vi "Lab Panel V5.23.vi"() -> ()   [LabVIEW 2013] (continued)
                          tunnel: w5914 -> [w5942 w5945]
                          tunnel: [w5942 w5944] -> w5912
                          frame False {
                          }
                          frame True {
                            n3204 = Multiply(x=w5946, y=w5945) -> (x*y=w5944:dbl)
                            n3205 = Multiply(x=w5946, y=w5948) -> (x*y=w5947:dbl)
                          }
                        }
                        n3206 = local read "SIG LAB04-2"() -> (w5931:T2)
                        n3207 = local read "SIG LAB04-1"() -> (w5933:T2)
                        n3208 = Bundle By Name(cluster=w5933, "Tmp Live"=w5913, "Tmp Neut"=w5912) -> (w5932:T2)
                        n3209 = Bundle By Name(cluster=w5931, "Tmp Live"=w5909, "Tmp Neut"=w5908) -> (w5930:T2)
                        n3210 = local write "SIG LAB04-1"(w5932) -> ()
                        n3211 = local write "SIG LAB04-2"(w5930) -> ()
                      }
                      frame 5.. {
                        n3212 = case shown="False" w5963 {
                          tunnel: [w5994 w5995] -> w5979
                          tunnel: w5962 -> [_ w5995]
                          frame False {
                            n3213 = local read "CAL LAB05"() -> (w5994:T14)
                          }
                          frame True {
                          }
                        }
                        n3214 = local read "LAB05 TEMP"() -> (w5969:T12)
                        n3215 = local read "TEMP LA05"() -> (w5970:T9)
                        n3216 = call "sub vi - temperature delay v3.vi"("2-run"=w5951, "1-run"=w5952, "temp values IN"=w5970, "temp signals"=w5969) -> ("T2-N"=w5965:dbl, "T2-L"=w5966:dbl, "T1-N"=w5967:dbl, "T1-L"=w5968:dbl, "temp values OUT"=w5964:T44)  [unwired: 3 in]
                        n3217 = local write "TEMP LA05"(w5964) -> ()
                        n3218 = Unbundle By Name(w5979) -> ("1 (TL) cal"=w5971:dbl, "1 (TN) cal"=w5974:dbl, "2 (TL) cal"=w5973:dbl, "2 (TN) cal"=w5972:dbl)  [unwired: 6 out]
                        n3219 = Multiply(x=w5968, y=w5971) -> (x*y=w5960:dbl)
                        n3220 = Multiply(x=w5967, y=w5974) -> (x*y=w5959:dbl)
                        n3221 = Multiply(x=w5966, y=w5973) -> (x*y=w5956:dbl)
                        n3222 = Multiply(x=w5965, y=w5972) -> (x*y=w5955:dbl)
                        n3223 = case shown="True" w5951 {
                          tunnel: w5956 -> [w5981 w5986]
                          tunnel: w5961 -> [_ w5984]
                          tunnel: [w5981 w5985] -> w5954
                          tunnel: w5955 -> [w5980 w5983]
                          tunnel: [w5980 w5982] -> w5953
                          frame False {
                          }
                          frame True {
                            n3224 = Multiply(x=w5984, y=w5983) -> (x*y=w5982:dbl)
                            n3225 = Multiply(x=w5984, y=w5986) -> (x*y=w5985:dbl)
                          }
                        }
                        n3226 = case shown="True" w5952 {
                          tunnel: w5960 -> [w5988 w5993]
                          tunnel: w5961 -> [_ w5991]
                          tunnel: [w5988 w5992] -> w5958
                          tunnel: w5959 -> [w5987 w5990]
                          tunnel: [w5987 w5989] -> w5957
                          frame False {
                          }
                          frame True {
                            n3227 = Multiply(x=w5991, y=w5990) -> (x*y=w5989:dbl)
                            n3228 = Multiply(x=w5991, y=w5993) -> (x*y=w5992:dbl)
                          }
                        }
                        n3229 = local read "SIG LAB05-1"() -> (w5978:T2)
                        n3230 = Bundle By Name(cluster=w5978, "Tmp Live"=w5958, "Tmp Neut"=w5957) -> (w5977:T2)
                        n3231 = local read "SIG LAB05-2"() -> (w5976:T2)
                        n3232 = Bundle By Name(cluster=w5976, "Tmp Live"=w5954, "Tmp Neut"=w5953) -> (w5975:T2)
                        n3233 = local write "SIG LAB05-1"(w5977) -> ()
                        n3234 = local write "SIG LAB05-2"(w5975) -> ()
                      }
                    }
                  }
                }
              }
            }
          }
          frame #20 {
            # "write data to display panel"
            n3235 = global write "Global display 1.vi" "TEST 5-2"(w6030) -> ()
            n3236 = global write "Global display 1.vi" "TEST 4-2"(w6032) -> ()
            n3237 = global write "Global display 1.vi" "TEST 1-2"(w6038) -> ()
            n3238 = global write "Global display 1.vi" "TEST 3-1"(w6035) -> ()
            n3239 = global write "Global display 1.vi" "TEST 5-1"(w6031) -> ()
            n3240 = global write "Global display 1.vi" "TEST 1-1"(w6039) -> ()
            n3241 = global write "Global display 1.vi" "TEST 3-2"(w6034) -> ()
            n3242 = global write "Global display 1.vi" "TEST 4-1"(w6033) -> ()
            n3243 = global write "Global display 1.vi" "TEST 2-2"(w6036) -> ()
            n3244 = global write "Global display 1.vi" "TEST 2-1"(w6037) -> ()
            n3245 = global read "Global display 3.vi" "log 1-1"() -> (→"LOG LAB01-1":string)
            n3246 = global read "Global display 3.vi" "log 3-1"() -> (→"LOG LAB03-1":string)
            n3247 = global read "Global display 3.vi" "log 1-2"() -> (→"LOG LAB01-2":string)
            n3248 = property on="Tab Control 2" class="TabCtl (strict)"() -> ("Pages"=w6029:refnum<vi>[])  [unwired: 2 in, 2 out]
            n3249 = global read "Global display 3.vi" "log 2-1"() -> (→"LOG LAB02-1":string)
            n3250 = global read "Global display 3.vi" "log 2-2"() -> (→"LOG LAB02-2":string)
            n3251 = global read "Global display 3.vi" "log 4-2"() -> (→"LOG LAB04-2":string)
            n3252 = global read "Global display 3.vi" "log 5-2"() -> (→"LOG LAB05-2":string)
            n3253 = global read "Global display 3.vi" "log 5-1"() -> (→"LOG LAB05-1":string)
            n3254 = global read "Global display 3.vi" "log 4-1"() -> (→"LOG LAB04-1":string)
            n3255 = global read "Global display 3.vi" "log 3-2"() -> (→"LOG LAB03-2":string)
            n3256 = Index Array(array=w6029, index=8) -> (element=w6027:refnum<vi>)
            n3257 = property class="Page"(reference=w6027) -> ("PageVis"=w6026:bool)  [unwired: 1 in, 2 out]
            n3258 = global write "Global display 3.vi" "admin"(w6026) -> ()
            n3259 = local read "O/I  LAB05-2"() -> (w6080:bool)
            n3260 = local read "O/I  LAB05-1"() -> (w6081:bool)
            n3261 = local read "O/I  LAB03-2"() -> (w6084:bool)
            n3262 = local read "O/I  LAB04-2"() -> (w6082:bool)
            n3263 = local read "O/I  LAB04-1"() -> (w6083:bool)
            n3264 = local read "O/I  LAB03-1"() -> (w6085:bool)
            n3265 = local read "O/I  LAB01-2"() -> (w6088:bool)
            n3266 = local read "O/I  LAB01-1"() -> (w6089:bool)
            n3267 = local read "O/I  LAB02-1"() -> (w6087:bool)
            n3268 = local read "O/I  LAB02-2"() -> (w6086:bool)
            n3269 = global write "Global display 1.vi" "5-2 O/F"(w6080) -> ()
            n3270 = global write "Global display 1.vi" "5-1 O/F"(w6081) -> ()
            n3271 = global write "Global display 1.vi" "4-1 O/F"(w6083) -> ()
            n3272 = global write "Global display 1.vi" "4-2 O/F"(w6082) -> ()
            n3273 = global write "Global display 1.vi" "3-2 O/F"(w6084) -> ()
            n3274 = global write "Global display 1.vi" "3-1 O/F"(w6085) -> ()
            n3275 = global write "Global display 1.vi" "2-2 O/F"(w6086) -> ()
            n3276 = global write "Global display 1.vi" "2-1 O/F"(w6087) -> ()
            n3277 = global write "Global display 1.vi" "1-2 O/F"(w6088) -> ()
            n3278 = global write "Global display 1.vi" "1-1 O/F"(w6089) -> ()
            n3279 = local read "TEMP START LAB02-2"() -> (w6012:cluster{"TL":dbl, "TN":dbl})
            n3280 = local read "run lab05-2"() -> (w6070:bool)
            n3281 = local read "TEMP START LAB01-2"() -> (w6014:cluster{"TL":dbl, "TN":dbl})
            n3282 = local read "TEMP START LAB02-1"() -> (w6013:cluster{"TL":dbl, "TN":dbl})
            n3283 = local read "TEMP START LAB04-1"() -> (w6009:cluster{"TL":dbl, "TN":dbl})
            n3284 = local read "TEMP START LAB04-2"() -> (w6008:cluster{"TL":dbl, "TN":dbl})
            n3285 = local read "run lab04-1"() -> (w6073:bool)
            n3286 = local read "run lab04-2"() -> (w6072:bool)
            n3287 = local read "run lab05-1"() -> (w6071:bool)
            n3288 = local read "TEMP START LAB01-1"() -> (w6015:cluster{"TL":dbl, "TN":dbl})
            n3289 = local read "TEMP START LAB05-2"() -> (w6006:cluster{"TL":dbl, "TN":dbl})
            n3290 = local read "TEMP START LAB05-1"() -> (w6007:cluster{"TL":dbl, "TN":dbl})
            n3291 = local read "run lab03-2"() -> (w6074:bool)
            n3292 = local read "TEMP START LAB03-2"() -> (w6010:cluster{"TL":dbl, "TN":dbl})
            n3293 = local read "TEMP START LAB03-1"() -> (w6011:cluster{"TL":dbl, "TN":dbl})
            n3294 = local read "run lab02-1"() -> (w6077:bool)
            n3295 = local read "run lab03-1"() -> (w6075:bool)
            n3296 = local read "run lab01-2"() -> (w6078:bool)
            n3297 = local read "run lab02-2"() -> (w6076:bool)
            n3298 = local read "run lab01-1"() -> (w6079:bool)
            n3299 = global write "Global display 1.vi" "5-2 R/S"(w6070) -> ()
            n3300 = global write "Global display 1.vi" "5-1 R/S"(w6071) -> ()
            n3301 = global write "Global display 1.vi" "4-2 R/S"(w6072) -> ()
            n3302 = global write "Global display 1.vi" "4-1 R/S"(w6073) -> ()
            n3303 = global write "Global display 1.vi" "3-2 R/S"(w6074) -> ()
            n3304 = global write "Global display 1.vi" "1-2 R/S"(w6078) -> ()
            n3305 = global write "Global display 1.vi" "2-1 R/S"(w6077) -> ()
            n3306 = global write "Global display 1.vi" "3-1 R/S"(w6075) -> ()
            n3307 = global write "Global display 1.vi" "2-2 R/S"(w6076) -> ()
            n3308 = global write "Global display 1.vi" "1-1 R/S"(w6079) -> ()
            n3309 = global write "Global display 3.vi" "TEMP ST 05-2"(w6006) -> ()
            n3310 = global write "Global display 3.vi" "TEMP ST 05-1"(w6007) -> ()
            n3311 = global write "Global display 3.vi" "TEMP ST 03-2"(w6010) -> ()
            n3312 = global write "Global display 3.vi" "TEMP ST 04-2"(w6008) -> ()
            n3313 = global write "Global display 3.vi" "TEMP ST 01-1"(w6015) -> ()
            n3314 = global write "Global display 3.vi" "TEMP ST 01-2"(w6014) -> ()
            n3315 = global write "Global display 3.vi" "TEMP ST 04-1"(w6009) -> ()
            n3316 = global write "Global display 3.vi" "TEMP ST 02-1"(w6013) -> ()
            n3317 = global write "Global display 3.vi" "TEMP ST 02-2"(w6012) -> ()
            n3318 = global write "Global display 3.vi" "TEMP ST 03-1"(w6011) -> ()
            n3319 = local read "DISP LAB04-2"() -> (w6062:T4)
            n3320 = local read "DISP LAB05-1"() -> (w6061:T4)
            n3321 = local read "DISP LAB04-1"() -> (w6063:T4)
            n3322 = local read "DISP LAB05-2"() -> (w6060:T4)
            n3323 = local read "DISP LAB03-1"() -> (w6065:T4)
            n3324 = local read "DISP LAB03-2"() -> (w6064:T4)
            n3325 = local read "DISP LAB01-2"() -> (w6068:T4)
            n3326 = local read "DISP LAB02-1"() -> (w6067:T4)
            n3327 = local read "DISP LAB02-2"() -> (w6066:T4)
            n3328 = local read "DISP LAB01-1"() -> (w6069:T4)
            n3329 = local read "TEMP RISE LAB05-1"() -> (w5997:cluster{"TL":dbl, "TN":dbl})
            n3330 = local read "TEMP RISE LAB05-2"() -> (w5996:cluster{"TL":dbl, "TN":dbl})
            n3331 = local read "TEMP RISE LAB04-2"() -> (w5998:cluster{"TL":dbl, "TN":dbl})
            n3332 = local read "TEMP RISE LAB04-1"() -> (w5999:cluster{"TL":dbl, "TN":dbl})
            n3333 = local read "TEMP RISE LAB03-2"() -> (w6000:cluster{"TL":dbl, "TN":dbl})
            n3334 = local read "TEMP RISE LAB03-1"() -> (w6001:cluster{"TL":dbl, "TN":dbl})
            n3335 = local read "TEMP RISE LAB01-2"() -> (w6004:cluster{"TL":dbl, "TN":dbl})
            n3336 = local read "TEMP RISE LAB02-2"() -> (w6002:cluster{"TL":dbl, "TN":dbl})
            n3337 = local read "TEMP RISE LAB01-1"() -> (w6005:cluster{"TL":dbl, "TN":dbl})
            n3338 = local read "TEMP RISE LAB02-1"() -> (w6003:cluster{"TL":dbl, "TN":dbl})
            n3339 = global write "Global display 2.vi" "DISP LAB05-1"(w6061) -> ()
            n3340 = global write "Global display 2.vi" "DISP LAB05-2"(w6060) -> ()
            n3341 = global write "Global display 2.vi" "DISP LAB04-2"(w6062) -> ()
            n3342 = global write "Global display 2.vi" "DISP LAB02-1"(w6067) -> ()
            n3343 = global write "Global display 2.vi" "DISP LAB02-2"(w6066) -> ()
            n3344 = global write "Global display 2.vi" "DISP LAB04-1"(w6063) -> ()
            n3345 = global write "Global display 2.vi" "DISP LAB01-2"(w6068) -> ()
            n3346 = global write "Global display 2.vi" "DISP LAB01-1"(w6069) -> ()
            n3347 = global write "Global display 2.vi" "DISP LAB03-1"(w6065) -> ()
            n3348 = global write "Global display 2.vi" "DISP LAB03-2"(w6064) -> ()
            n3349 = global write "Global display 3.vi" "TEMP RS 05-2"(w5996) -> ()
            n3350 = global write "Global display 3.vi" "TEMP RS 05-1"(w5997) -> ()
            n3351 = global write "Global display 3.vi" "TEMP RS 03-2"(w6000) -> ()
            n3352 = global write "Global display 3.vi" "TEMP RS 02-1"(w6003) -> ()
            n3353 = global write "Global display 3.vi" "TEMP RS 02-2"(w6002) -> ()
            n3354 = global write "Global display 3.vi" "TEMP RS 04-2"(w5998) -> ()
            n3355 = global write "Global display 3.vi" "TEMP RS 01-2"(w6004) -> ()
            n3356 = global write "Global display 3.vi" "TEMP RS 03-1"(w6001) -> ()
            n3357 = global write "Global display 3.vi" "TEMP RS 04-1"(w5999) -> ()
            n3358 = global write "Global display 3.vi" "TEMP RS 01-1"(w6005) -> ()
            n3359 = local read "SET LAB05-2"() -> (w6050:T5)
            n3360 = local read "SET LAB05-1"() -> (w6051:T5)
            n3361 = local read "SET LAB04-1"() -> (w6053:T5)
            n3362 = local read "SET LAB04-2"() -> (w6052:T5)
            n3363 = local read "SET LAB03-1"() -> (w6055:T5)
            n3364 = local read "SET LAB03-2"() -> (w6054:T5)
            n3365 = local read "SET LAB02-2"() -> (w6056:T5)
            n3366 = local read "SET LAB01-2"() -> (w6058:T5)
            n3367 = local read "SET LAB02-1"() -> (w6057:T5)
            n3368 = local read "SET LAB01-1"() -> (w6059:T5)
            n3369 = global write "Global display 2.vi" "SET LAB05-2"(w6050) -> ()
            n3370 = global write "Global display 2.vi" "SET LAB05-1"(w6051) -> ()
            n3371 = global write "Global display 2.vi" "SET LAB04-1"(w6053) -> ()
            n3372 = global write "Global display 2.vi" "SET LAB04-2"(w6052) -> ()
            n3373 = global write "Global display 2.vi" "SET LAB03-2"(w6054) -> ()
            n3374 = global write "Global display 2.vi" "SET LAB02-2"(w6056) -> ()
            n3375 = global write "Global display 2.vi" "SET LAB03-1"(w6055) -> ()
            n3376 = global write "Global display 2.vi" "SET LAB01-2"(w6058) -> ()
            n3377 = global write "Global display 2.vi" "SET LAB01-1"(w6059) -> ()
            n3378 = global write "Global display 2.vi" "SET LAB02-1"(w6057) -> ()
            n3379 = local read "RESULT LAB01-1"() -> (w6049:bool)
            n3380 = local read "RESULT LAB03-2"() -> (w6044:bool)
            n3381 = local read "RESULT LAB04-1"() -> (w6043:bool)
            n3382 = local read "RESULT LAB04-2"() -> (w6042:bool)
            n3383 = local read "RESULT LAB02-2"() -> (w6046:bool)
            n3384 = local read "RESULT LAB01-2"() -> (w6048:bool)
            n3385 = local read "RESULT LAB02-1"() -> (w6047:bool)
            n3386 = local read "RESULT LAB03-1"() -> (w6045:bool)
            n3387 = local read "RESULT LAB05-1"() -> (w6041:bool)
            n3388 = local read "RESULT LAB05-2"() -> (w6040:bool)
            n3389 = global write "Global display 2.vi" "RESULT LAB05-1"(w6041) -> ()
            n3390 = global write "Global display 2.vi" "RESULT LAB01-2"(w6048) -> ()
            n3391 = global write "Global display 2.vi" "RESULT LAB03-2"(w6044) -> ()
            n3392 = global write "Global display 2.vi" "RESULT LAB04-1"(w6043) -> ()
            n3393 = global write "Global display 2.vi" "RESULT LAB04-2"(w6042) -> ()
            n3394 = global write "Global display 2.vi" "RESULT LAB05-2"(w6040) -> ()
            n3395 = global write "Global display 2.vi" "RESULT LAB03-1"(w6045) -> ()
            n3396 = global write "Global display 2.vi" "RESULT LAB02-1"(w6047) -> ()
            n3397 = global write "Global display 2.vi" "RESULT LAB02-2"(w6046) -> ()
            n3398 = global write "Global display 2.vi" "RESULT LAB01-1"(w6049) -> ()
          }
          frame #21 {
            # "simulate values"
            n3399 = global write "Global display 4.vi" "LAB deg C"("LAB deg C") -> ()
          }
          frame #22 {
            # "end main and display program"
            n3400 = stacked-sequence {
              seq-local: [_ w6094 _] -> [_ _ w6097]
              tunnel: w6091 -> [w6092 _ _]
              frame #0 {
                n3401 = case shown="True" w6092 {
                  frame False {
                  }
                  frame True {
                    n3402 = One Button Dialog(message="Excessive number of USB \nresets done, re-start program.") -> ()  [unwired: 1 in, 1 out]
                  }
                }
              }
              frame #1 {
                # "check for reset error"
                n3403 = local read "Reset Error"() -> (w6094:bool)
                n3404 = case shown="True" w6094 {
                  frame False {
                  }
                  frame True {
                    n3405 = One Button Dialog(message="USB Reset ERROR, program will be stopped.\nClose program, close windows, switch panel off\nand re power panel. If error persists seek help.") -> ()  [unwired: 1 in, 1 out]
                  }
                }
              }
              frame #2 {
                # "end labview session"
                n3406 = Or(x=w6097, y="stop all") -> (x .or. y?=w6096:bool)
                n3407 = Quit LabVIEW(quit? (T)=w6096) -> ()
                n3408 = global write "Global display 1.vi" "stop disp"(w6096) -> ()
              }
            }
          }
        }
        n3409 = node-c288() -> ()  [unwired: 1 in, 1 out]
        "loops" <- w335
      }
      n3410 = node-c288(w308) -> ()  [unwired: 1 out]
    }
  }
